vi "Simple Spectrometer.vi"() -> ()   [LabVIEW 2013]
uses:
  lightfield-automation-labview/LightField Automation.lvclass
panel:
  in  "ExperimentName":string
  in  "stop":bool
  in  "Center Wavelength":dbl
  in  "Grating":string(combo)
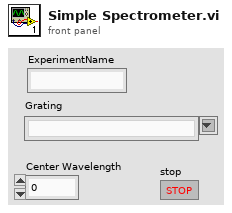
[diagram p1: front panel]
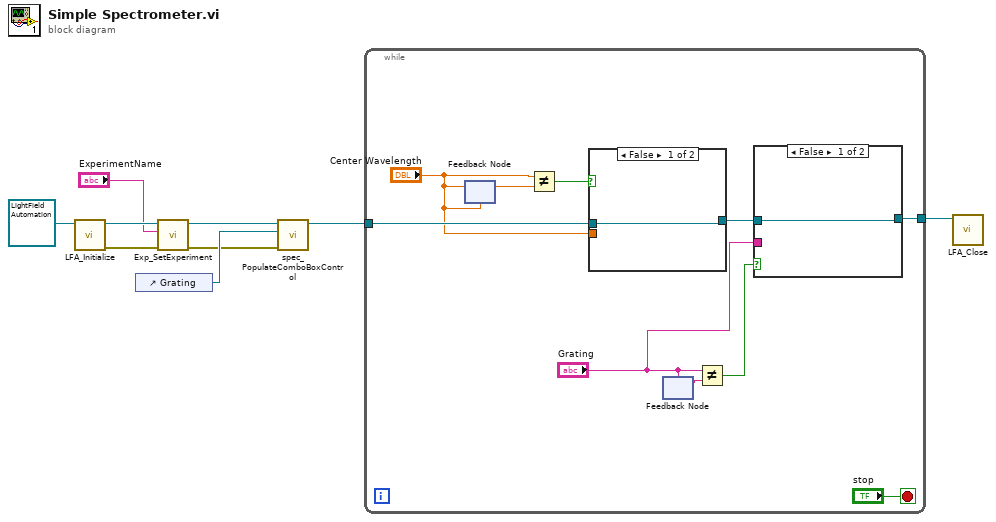
[diagram p0: block diagram]
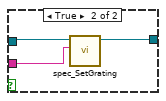
[diagram p2: hidden frame]
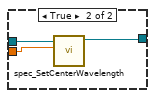
[diagram p3: hidden frame]
diagram:
  n1 = call "LFA_Initialize.vi"("LightField Automation in"=refnum<class "LightField Automation.lvclass"> refnum ("LightField Automation.lvclass")) -> ("error out"=w5:errorcluster, "LightField Automation out"=w6:refnum<class "LightField Automation.lvclass">)  [unwired: 9 in]
  n2 = control-ref of="Grating"() -> (w9:refnum<vi>)
  n3 = call "Exp_SetExperiment.vi"("error in (no error)"=w5, "ExperimentName"="ExperimentName", "LightField Automation in"=w6) -> ("error out"=w3:errorcluster, "LightField Automation out"=w2:refnum<class "LightField Automation.lvclass">)  [unwired: 7 in]
  n4 = call "spec_PopulateComboBoxControl.vi"("error in (no error)"=w3, "Combo Box Reference"=w9, "LightField Automation in"=w2) -> ("LightField Automation out"=w8:refnum<class "LightField Automation.lvclass">)  [unwired: 7 in, 1 out]
  n5 = while {
    tunnel: w8 -> [w15]
    tunnel: [w10] -> w1
    stop <- "stop" stop-if-true
    n6 = feedback-in #1("Center Wavelength") -> ()
    n7 = feedback #1("Center Wavelength") -> (w19:dbl)
    n8 = Not Equal?(x="Center Wavelength", y=w19) -> (x != y?=w17:bool)
    n9 = case shown="False" w17 {
      tunnel: w15 -> [w24 w27]
      tunnel: [w24 w26] -> w13
      tunnel: "Center Wavelength" -> [_ w25]
      frame False {
      }
      frame True {
        n10 = call "spec_SetCenterWavelength.vi"("Center Wavelength"=w25, "LightField Automation in"=w27) -> ("LightField Automation out"=w26:refnum<class "LightField Automation.lvclass">)  [unwired: 8 in, 1 out]
      }
    }
    n11 = feedback #2("Grating") -> (w18:string)
    n12 = feedback-in #2("Grating") -> ()
    n13 = Not Equal?(x="Grating", y=w18) -> (x != y?=w16:bool)
    n14 = case shown="False" w16 {
      tunnel: "Grating" -> [_ w23]
      tunnel: w13 -> [w20 w22]
      tunnel: [w20 w21] -> w10
      frame False {
      }
      frame True {
        n15 = call "spec_SetGrating.vi"("GratingSelected"=w23, "LightField Automation in"=w22) -> ("LightField Automation out"=w21:refnum<class "LightField Automation.lvclass">)  [unwired: 8 in, 1 out]
      }
    }
  }
  n16 = call "LFA_Close.vi"("LightField Automation in"=w1) -> ()  [unwired: 9 in, 2 out]
